vi "LOGIC_SendError.vi"(8 "error in (no error)":errorcluster, 9 "log file":path, 10 "message":string) -> (0 "error out":errorcluster)   [LabVIEW 2016]
uses:
  Common/public/vis/CMN_FVAR_action.ctl
  LOGIC_gbls.vi
  DBSHAND/private/vis/DatabaseHand_Element_Set(string).vi
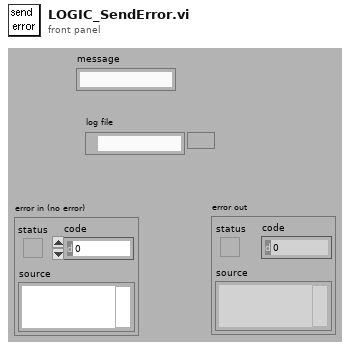
[diagram p1: front panel]
types:
  T1 = typedef "CMN_FVAR_action.ctl" = enum16{"read", "write"}
  T2 = typedef "DatabaseHand_RefNum.ctl" = refnum<vi>
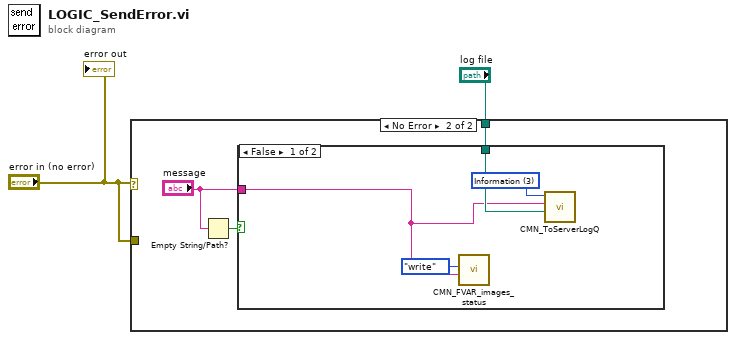
[diagram p0: block diagram]
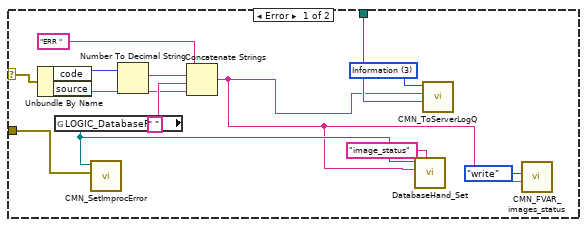
[diagram p2: hidden frame]
diagram:
  n1 = case shown="No Error" "error in (no error)" {
    selector: "error in (no error)" -> [w14 _]
    tunnel: "log file" -> [w8 w18]
    tunnel: "error in (no error)" -> [w7 _]
    frame Error {
      w15 = u16 3 items=["command", "imediateReply", "Callback Reply", "Information"] ("type")
      n2 = Unbundle By Name(w14) -> ("code"=w12:i32, "source"=w9:string)
      n3 = global read "LOGIC_gbls.vi" "LOGIC_DatabaseRef"() -> (w5:T2)
      n4 = call "CMN_SetImprocError.vi"("improc error"=w7, "Database RefNum in"=w5) -> ()  [unwired: 1 in, 9 out]
      n5 = Number To Decimal String(number=w12) -> (decimal integer string=w11:string)  [unwired: 1 out]
      n6 = Concatenate Strings("ERR ", w11, " ", w9) -> (w3:string)
      n7 = call-poly "DatabaseHand_Set.vi"("name"="image_status", "value"=w3, "Database RefNum in"=w5) -> ()  [unwired: 5 in, 4 out]
      n8 = call "CMN_ToServerLogQ.vi"("file"=w8, "string"=w3, "type"=w15) -> ()  [unwired: 3 in, 5 out]
      n9 = call "CMN_FVAR_images_status.vi"("value in"=w3, "action"=CMN_FVAR_action."write") -> ()  [unwired: 9 out]
    }
    frame No Error {
      n10 = Empty String/Path?(string/path="message") -> (empty?=w16:bool)
      n11 = case shown="False" w16 {
        tunnel: w18 -> [w21 _]
        tunnel: "message" -> [w20 _]
        frame False {
          w22 = u16 3 items=["command", "imediateReply", "Callback Reply", "Information"] ("type")
          n12 = call "CMN_FVAR_images_status.vi"("value in"=w20, "action"=CMN_FVAR_action."write") -> ()  [unwired: 9 out]
          n13 = call "CMN_ToServerLogQ.vi"("file"=w21, "string"=w20, "type"=w22) -> ()  [unwired: 3 in, 5 out]
        }
        frame True {
        }
      }
    }
  }
  "error out" <- "error in (no error)"
